vi "compatOverwrite.vi"(1 "overwrite (F)":bool) -> (0 "overwrite?":T1(ring))   [LabVIEW 2020]
doc: "Used in conjunction with Open/Create/Replace File to get the correct operation mode depending on whether or not the file should be overwritten."
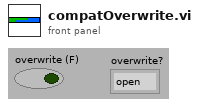
[diagram p1: front panel]
types:
  T1 = enum16{"open", "replace", "create", "open or create", "replace or create", "replace or create with confirmation"}
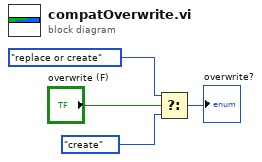
[diagram p0: block diagram]
diagram:
  n1 = Select(t=T1."replace or create" ("operation (0:open)"), s="overwrite (F)", f=T1."create" ("operation (0:open)")) -> (s? t:f=→"overwrite?":T1)
